vi "Create State Data.vi"(8 "error in (no error)":errorcluster) -> (0 "error out":errorcluster, 3 "Process State Data out":refnum<data-value>)   [LabVIEW 2022 SP3, in "Process State Data.lvclass"]
uses:
  Process State Data.lvclass
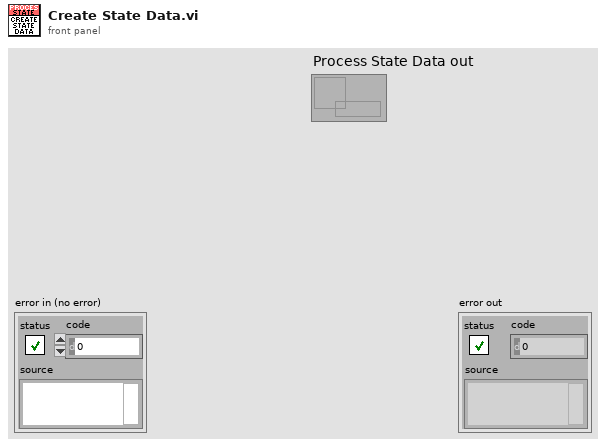
[diagram p1: front panel]
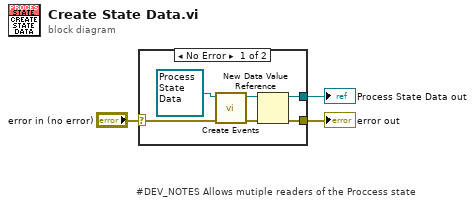
[diagram p0: block diagram]
diagram:
  # "#DEV_NOTES Allows mutiple readers of the Proccess state"
  n1 = case shown="No Error" "error in (no error)" {
    selector: "error in (no error)" -> [w5 w10]
    tunnel: [w8 w10] -> w2
    tunnel: [w9 _] -> w1
    frame No Error {
      n2 = call "Create Events.vi"("error in (no error)"=w5, "Process State Data in"=refnum<class "Process State Data.lvclass"> refnum) -> ("error out"=w4:errorcluster, "Process State Data out"=w6:refnum<class "Process State Data.lvclass">)  [unwired: 8 in]
      n3 = New Data Value Reference(data value=w6, error in=w4) -> (data value reference=w9:refnum<data-value>, error out=w8:errorcluster)
    }
    frame Error {
    }
  }
  "error out" <- w2
  "Process State Data out" <- w1
